vi "CREATE_INITIAL_STRING.vi"(9 "appended array":string[](array[string]), 11 "String in":string) -> (3 "String out":string)   [LabVIEW 2016]
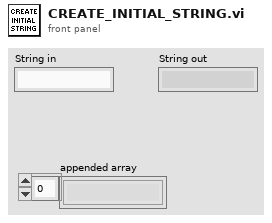
[diagram p1: front panel]
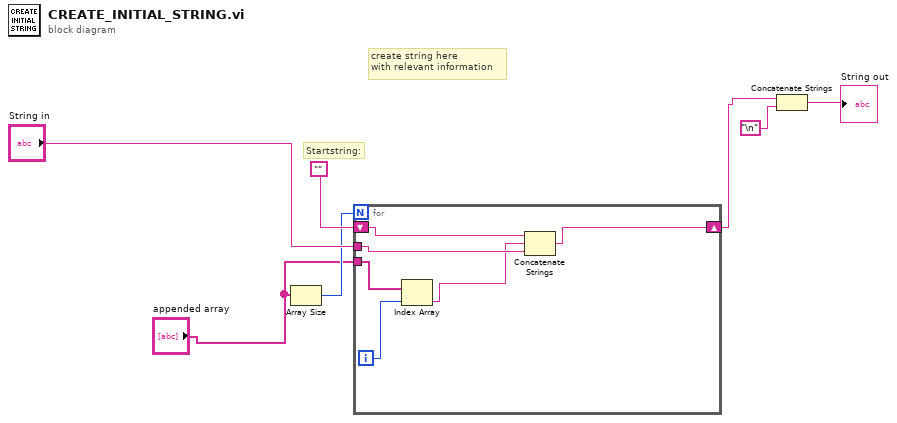
[diagram p0: block diagram]
diagram:
  # "Startstring:"
  # "create string here \nwith relevant information"
  n1 = Array Size(array="appended array") -> (size(s)=w5:i32)
  n2 = for {
    N: w5 -> [_]
    tunnel: "appended array" -> [w12]
    tunnel: "String in" -> [w11]
    shift-right: [w9] -> w3
    shift-left: "" -> [w10]
    i -> [w13]
    n3 = Index Array(array=w12, index=w13) -> (element=w8:string)
    n4 = Concatenate Strings(w10, w8, w11) -> (w9:string)
  }
  n5 = Concatenate Strings(w3, "\n" ("End of Line Constant")) -> (→"String out":string)
